vi "ScopePitcher.vi"() -> ()   [LabVIEW 2012]
uses:
  <instrlib>/niScope/Controls/niScope vertical coupling.ctl
  <instrlib>/niScope/Configure/Trigger/niScope Configure Trigger Edge.vi
  <instrlib>/niScope/Acquire/Fetch/niScope Multi Fetch Cluster.vi
panel:
  in  "stop":bool
  in  "Signal Coupling":T1=1 caption="vertical coupling" items=["AC", "DC", "Ground"]
  in  "Reference Position (%)":dbl=50.0 caption="Reference Position" format="%.1f"
  out "Total Acquisition Time (s)":dbl
  in  "Timebase":dbl(ring)=1e-05 items=["100ns"=1e-07, "1us"=1e-06, "10us"=1e-05, "100us"=0.0001, "1ms"=0.001, "10ms"=0.01, "100ms"=0.1]
  in  "Trigger Level":dbl=2.0 format="%.2f"
  in  "Number of Samples":i32=1000
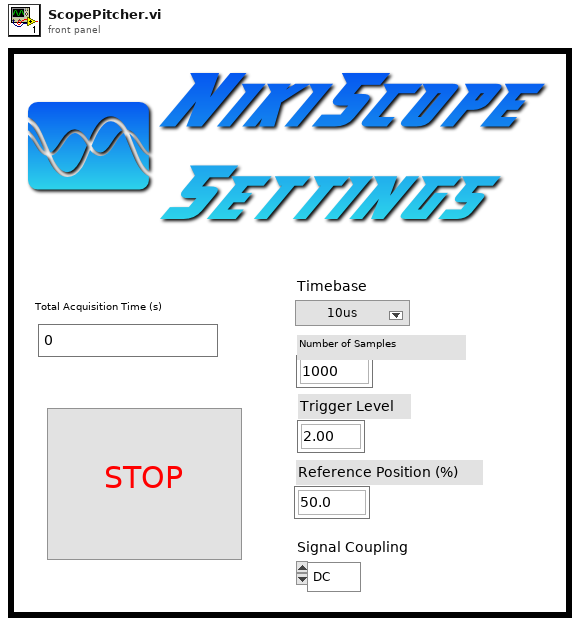
[diagram p1: front panel]
types:
  T1 = typedef "niScope vertical coupling.ctl" = i32
  T2 = cluster{"relativeInitialX":dbl, "xIncrement":dbl, "wfm":dbl[]}[]
  T3 = cluster{"relativeInitialX":dbl, "xIncrement":dbl, "wfm":dbl[]}
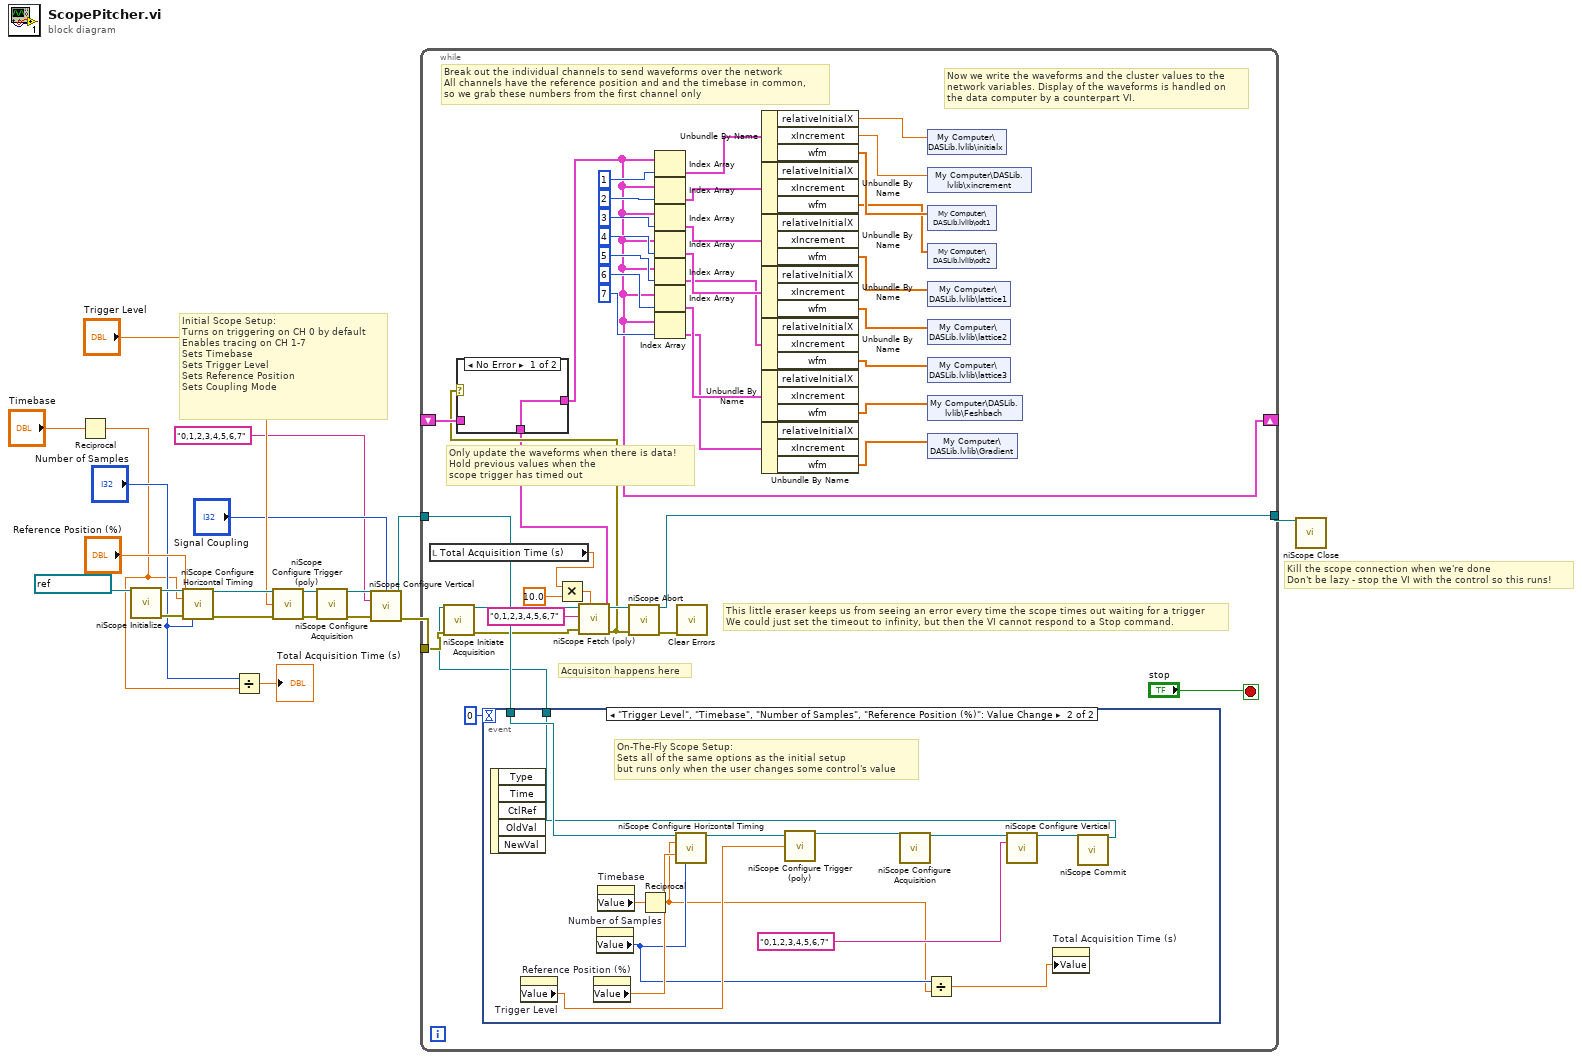
[diagram p0: block diagram]
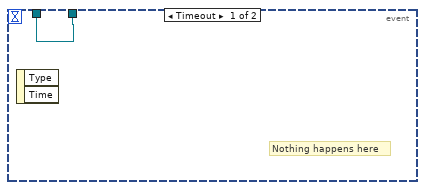
[diagram p3: hidden frame]
diagram:
  # "Kill the scope connection when we're done\nDon't be lazy - stop the VI with the control so this runs!"
  # "Initial Scope Setup:\nTurns on triggering on CH 0 by default\nEnables tracing on CH 1-7\nSets Timebase\nSets Trigger Level\nSets Reference Position\nSets Coupling Mode"
  n1 = Reciprocal(x="Timebase") -> (1/x=w1:dbl)
  n2 = call <instrlib>:"niScope Initialize.vi"("resource name"=refnum<k15> "PXI1Slot4") -> ("instrument handle"=w19:refnum<k15>, "error out"=w18:errorcluster)  [unwired: 13 in]
  n3 = call <instrlib>:"niScope Configure Horizontal Timing.vi"("instrument handle"=w19, "min sample rate"=w1, "reference position"="Reference Position (%)", "error in"=w18, "min record length"="Number of Samples") -> ("instrument handle out"=w17:refnum<k15>, "error out"=w8:errorcluster)  [unwired: 9 in]
  n4 = Divide(x="Number of Samples", y=w1) -> (x/y=→"Total Acquisition Time (s)":dbl)
  n5 = call-poly <instrlib>:"niScope Configure Trigger (poly).vi"("instrument handle"=w17, "trigger level"="Trigger Level", "error in"=w8) -> ("instrument handle out"=w14:refnum<k15>, "error out"=w13:errorcluster)  [unwired: 11 in]
  n6 = call <instrlib>:"niScope Configure Acquisition.vi"("instrument handle"=w14, "error in"=w13) -> ("instrument handle out"=w11:refnum<k15>, "error out"=w12:errorcluster)  [unwired: 12 in]
  n7 = call <instrlib>:"niScope Configure Vertical.vi"("instrument handle"=w11, "vertical coupling"="Signal Coupling", "channels"="0,1,2,3,4,5,6,7", "error in"=w12) -> ("instrument handle out"=w15:refnum<k15>, "error out"=w10:errorcluster)  [unwired: 10 in]
  n8 = while {
    tunnel: w15 -> [w58]
    tunnel: w10 -> [w57]
    tunnel: [w61] -> w9
    shift-right: [w34] -> _
    shift-left: _ -> [w45]
    stop <- "stop" stop-if-true
    # "Now we write the waveforms and the cluster values to the\nnetwork variables. Display of the waveforms is handled on\nthe data computer by a counterpart VI."
    # "This little eraser keeps us from seeing an error every time the scope times out waiting for a trigger\nWe could just set the timeout to infinity, but then the VI cannot respond to a Stop command."
    # "Break out the individual channels to send waveforms over the network\nAll channels have the reference position and and the timebase in common,\nso we grab these numbers from the first channel only"
    # "Only update the waveforms when there is data!\nHold previous values when the \nscope trigger has timed out"
    # "Acquisiton happens here"
    n9 = local read "Total Acquisition Time (s)"() -> (w23:dbl)
    n10 = event shown="[1] \"Trigger Level\", \"Timebase\", \"Number of Samples\", \"Reference Position (%)\": Value Change" {
      selector: _ -> [_ _]
      dyn-events: _ -> [_ _]
      timeout: 0 -> [_ _]
      tunnel: w58 -> [w64 w77]
      tunnel: [w64 w66] -> w53
      event Timeout {
        # "Nothing happens here"
        n11 = event-data() -> ()  [unwired: 1 in, 2 out]
      }
      event "Trigger Level", "Timebase", "Number of Samples", "Reference Position (%)": Value Change {
        # "On-The-Fly Scope Setup:\nSets all of the same options as the initial setup\nbut runs only when the user changes some control's value"
        n12 = event-data() -> ()  [unwired: 1 in, 5 out]
        n13 = property on="Trigger Level" class="DigNum (strict)"() -> ("Value"=w72:dbl)  [unwired: 2 in, 2 out]
        n14 = property on="Reference Position (%)" class="DigNum (strict)"() -> ("Value"=w73:dbl)  [unwired: 2 in, 2 out]
        n15 = property on="Number of Samples" class="DigNum (strict)"() -> ("Value"=w68:i32)  [unwired: 2 in, 2 out]
        n16 = property on="Timebase" class="Ring (strict)"() -> ("Value"=w71:dbl)  [unwired: 2 in, 2 out]
        n17 = Reciprocal(x=w71) -> (1/x=w65:dbl)
        n18 = call <instrlib>:"niScope Configure Horizontal Timing.vi"("instrument handle"=w77, "min sample rate"=w65, "reference position"=w73, "min record length"=w68) -> ("instrument handle out"=w76:refnum<k15>)  [unwired: 10 in, 1 out]
        n19 = call-poly <instrlib>:"niScope Configure Trigger (poly).vi"("instrument handle"=w76, "trigger level"=w72) -> ("instrument handle out"=w75:refnum<k15>)  [unwired: 12 in, 1 out]
        n20 = call <instrlib>:"niScope Configure Acquisition.vi"("instrument handle"=w75) -> ("instrument handle out"=w74:refnum<k15>)  [unwired: 13 in, 1 out]
        n21 = Divide(x=w68, y=w65) -> (x/y=w70:dbl)
        n22 = call <instrlib>:"niScope Configure Vertical.vi"("instrument handle"=w74, "channels"="0,1,2,3,4,5,6,7") -> ("instrument handle out"=w69:refnum<k15>)  [unwired: 12 in, 1 out]
        n23 = property on="Total Acquisition Time (s)" class="DigNum (strict)"("Value"=w70) -> ()  [unwired: 2 in, 2 out]
        n24 = call <instrlib>:"niScope Commit.vi"("instrument handle"=w69) -> ("instrument handle out"=w66:refnum<k15>)  [unwired: 13 in, 1 out]
      }
    }
    n25 = call <instrlib>:"niScope Initiate Acquisition.vi"("instrument handle"=w53, "error in"=w57) -> ("instrument handle out"=w56:refnum<k15>, "error out"=w55:errorcluster)  [unwired: 12 in]
    n26 = Multiply(x=w23, y=10.0) -> (x*y=w22:dbl)
    n27 = call-poly <instrlib>:"niScope Fetch (poly).vi"("timeout"=w22, "error in"=w55, "channels"="0,1,2,3,4,5,6,7", "instrument handle"=w56) -> ("error out"=w44:errorcluster, "waveform"=w43:T2, "instrument handle out"=w54:refnum<k15>)  [unwired: 4 in, 1 out]
    n28 = case shown="No Error" w44 {
      tunnel: w45 -> [_ w63]
      tunnel: [w62 w63] -> w34
      tunnel: w43 -> [w62 _]
      frame No Error {
      }
      frame Error {
      }
    }
    n29 = call <instrlib>:"niScope Abort.vi"("instrument handle"=w54, "error in"=w44) -> ("instrument handle out"=w61:refnum<k15>, "error out"=w60:errorcluster)  [unwired: 12 in]
    n30 = Index Array(array=w34, index=1) -> (element=w41:T3)
    n31 = Index Array(array=w34, index=2) -> (element=w40:T3)
    n32 = Index Array(array=w34, index=3) -> (element=w39:T3)
    n33 = Index Array(array=w34, index=4) -> (element=w38:T3)
    n34 = Index Array(array=w34, index=5) -> (element=w37:T3)
    n35 = Index Array(array=w34, index=6) -> (element=w36:T3)
    n36 = Index Array(array=w34, index=7) -> (element=w33:T3)
    n37 = call <vilib>:"Clear Errors.vi"("error in (no error)"=w60) -> ()  [unwired: 6 in, 1 out]
    n38 = Unbundle By Name(w41) -> ("relativeInitialX"=w32:dbl, "xIncrement"=w31:dbl, "wfm"=w30:dbl[])
    n39 = Unbundle By Name(w40) -> ("wfm"=w29:dbl[])  [unwired: 2 out]
    n40 = Unbundle By Name(w39) -> ("wfm"=w28:dbl[])  [unwired: 2 out]
    n41 = Unbundle By Name(w38) -> ("wfm"=w27:dbl[])  [unwired: 2 out]
    n42 = Unbundle By Name(w37) -> ("wfm"=w26:dbl[])  [unwired: 2 out]
    n43 = Unbundle By Name(w36) -> ("wfm"=w25:dbl[])  [unwired: 2 out]
    n44 = Unbundle By Name(w33) -> ("wfm"=w24:dbl[])  [unwired: 2 out]
    n45 = shared-variable "My Computer\\DASLib.lvlib\\initialx"(w32) -> ()  [unwired: 1 in, 1 out]
    n46 = shared-variable "My Computer\\DASLib.lvlib\\xincrement"(w31) -> ()  [unwired: 1 in, 1 out]
    n47 = shared-variable "My Computer\\DASLib.lvlib\\odt1"(w30) -> ()  [unwired: 1 in, 1 out]
    n48 = shared-variable "My Computer\\DASLib.lvlib\\odt2"(w29) -> ()  [unwired: 1 in, 1 out]
    n49 = shared-variable "My Computer\\DASLib.lvlib\\lattice1"(w28) -> ()  [unwired: 1 in, 1 out]
    n50 = shared-variable "My Computer\\DASLib.lvlib\\lattice2"(w27) -> ()  [unwired: 1 in, 1 out]
    n51 = shared-variable "My Computer\\DASLib.lvlib\\lattice3"(w26) -> ()  [unwired: 1 in, 1 out]
    n52 = shared-variable "My Computer\\DASLib.lvlib\\Feshbach"(w25) -> ()  [unwired: 1 in, 1 out]
    n53 = shared-variable "My Computer\\DASLib.lvlib\\Gradient"(w24) -> ()  [unwired: 1 in, 1 out]
  }
  n54 = call <instrlib>:"niScope Close.vi"("instrument handle"=w9) -> ()  [unwired: 14 in, 1 out]
